vi "Master_DARPA.vi"() -> ()   [LabVIEW 2021]
uses:
  Control 2.ctl
  Settings.ctl
  <vilib>/DAQmx/write.llb/DAQmx Write (Analog DBL 1Chan 1Samp).vi
  <vilib>/DAQmx/write.llb/DAQmx Write (Analog Wfm 1Chan NSamp).vi
  <vilib>/DAQmx/write.llb/DAQmx Write (Digital 1D U32 1Chan NSamp).vi
  <vilib>/DAQmx/read.llb/DAQmx Read (Counter DBL 1Chan 1Samp).vi
  <vilib>/DAQmx/create/channels.llb/DAQmx Create Channel (AO-Voltage-Basic).vi
  <vilib>/DAQmx/create/channels.llb/DAQmx Create Channel (CI-Count Edges).vi
  <vilib>/DAQmx/miscellaneous.llb/DAQmx Fill In Error Info.vi
  <vilib>/DAQmx/create/channels.llb/DAQmx Create Channel (DO-Digital Output).vi
  <vilib>/DAQmx/configure/timing.llb/DAQmx Timing (Sample Clock).vi
  <resource>/objmgr/daqmx.rc
panel:
  out "s per ch":T1 format="%#_9f"
  out "Trial End Signal":bool
  in  "stop":bool
  in  "Blue Exposure Width [50-100] (ms)":T1=41.0 format="%#_9f"
  in  "Amber Start Time":T1=60.0 format="%#_9f"
  in  "Red Start (ms)":T1=120.0 format="%#_9f"
  in  "Red Exposure Width (ms)":T1=41.0 format="%#_9f"
  in  "Amber Exposure Width (ms)":T1=41.0 format="%#_9f"
  in  "base path":path=path "E:/DARPA/MW-LSCI1/5_14_22"
  in  "Delay end (ms)":dbl=102.0
  out "Stimulation":bool
  in  "AOM Voltage":dbl=0.085 format="%0.3f"
  out "String 7":string="AOM Settings"
  out "String 6":string="Stroke Settings"
  out "String 5":string="Intrinsic Imaging"
  in  "LED 625 nm":bool
  in  "LED 580 nm":bool
  out "Trial #":i32=2
  out "Frames acquired":dbl=576.0 format="%0.2f"
  out "Number of Samples (Total)":dbl=18000.0
  out "Period (ms)":dbl=6.5
  out "String 4":string="Experimental Summary"
  out "String 3":string="Stimulation Control"
  out "String 2":string="Sequence Control"
  out "String":string="Trials Control"
  in  "Strength (V)":dbl=10.0
  in  "# of stimulations":i32=2
  in  "Delay (ms)":dbl=35.0
  in  "Width of pulse (ms)":dbl=60.0
  in  "# of Sequences":dbl=750.0
  in  "Sampling Rate (Hz)":T1=100000.0 format="%#_9f"
  in  "Frames/Seq":i32=12
  in  "Exposure Width (ms)":T1=5.0 format="%#_9f"
  in  "Time Between (ms)":T2=1.5 format="%#_9f"
  in  "Pre-stimulus Time":dbl=30.0 format="%.6f"
  in  "Time b/w Trials (s)":dbl=10.0 caption="Delay Time (s)"
  in  "# Trials":i32=5
  in  "Time domain signal":T3(tab)
  out "LSCI Sequence":cluster{i32, dbl, dbl[]}(graph)={0, 1e-05, array[18000 elements]}
  out "Red LED":cluster{i32, dbl, dbl[]}(graph)={0, 1e-05, array[18000 elements]}
  out "Amber LED":cluster{i32, dbl, dbl[]}(graph)={0, 1e-05, array[18000 elements]}
  out "Blue LED":cluster{i32, dbl, dbl[]}(graph)={0, 1e-05, array[18000 elements]}
  out "EMCCD":cluster{i32, dbl, dbl[]}(graph)={0, 1e-05, array[18000 elements]}
  out "Whisker Cam":cluster{i32, dbl, dbl[]}(graph)={0, 1e-05, array[18000 elements]}
  out "Whisker Stim":cluster{i32, dbl, dbl[]}(graph)={0, 1e-05, array[18000 elements]}
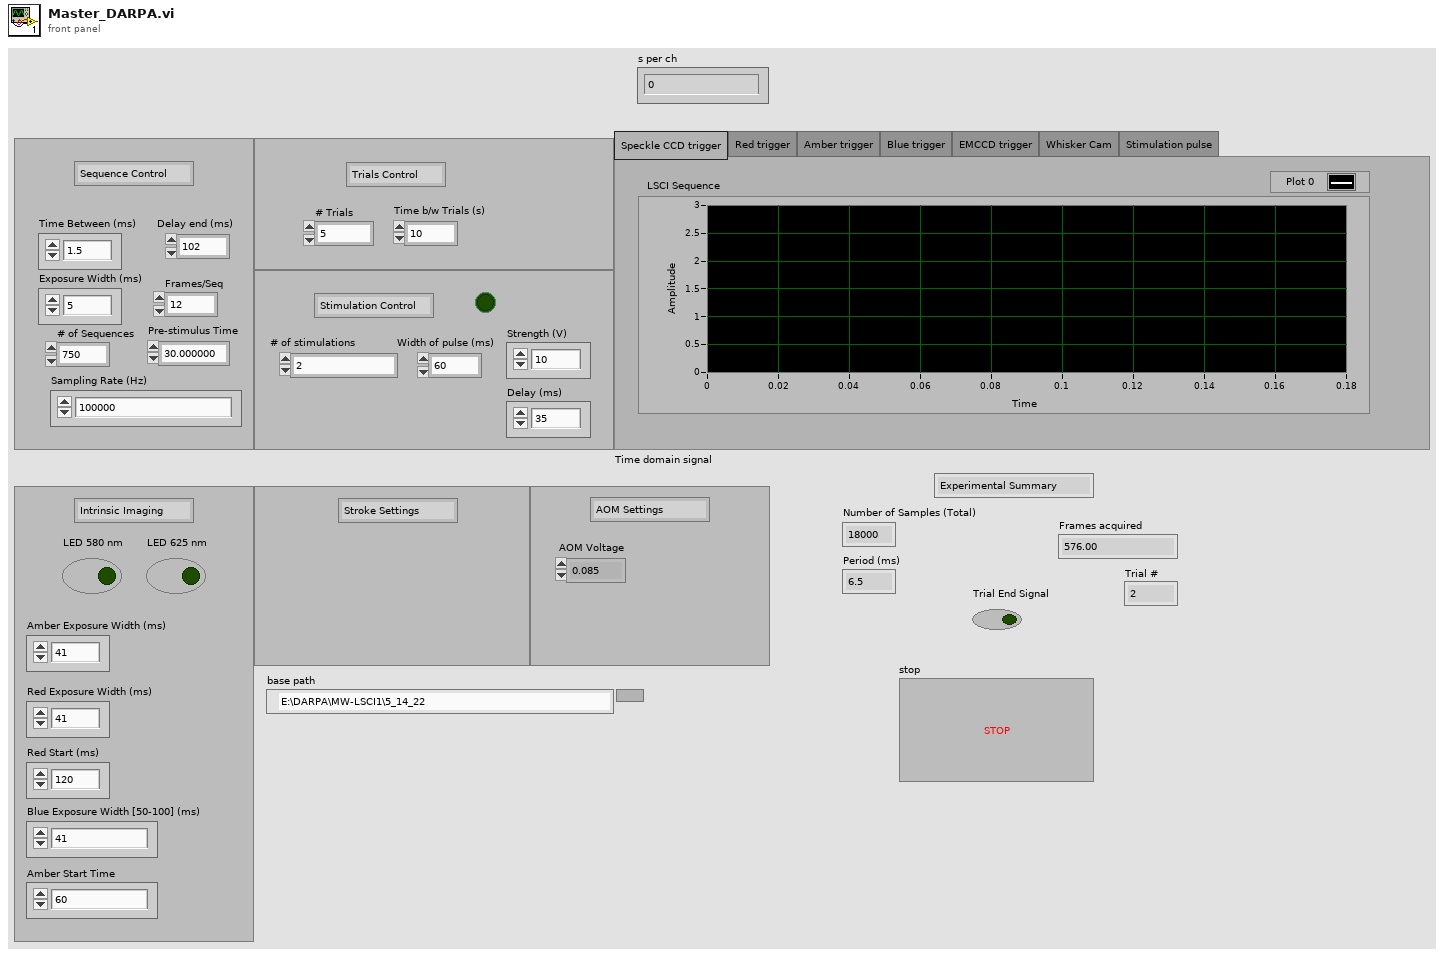
[diagram p1: front panel]
types:
  T1 = typedef "Settings.ctl" = dbl
  T2 = typedef "Control 2.ctl" = dbl
  T3 = enum32{"Speckle CCD trigger", "Red trigger", "Amber trigger", "Blue trigger", "EMCCD trigger", "Whisker Cam", "Stimulation pulse"}
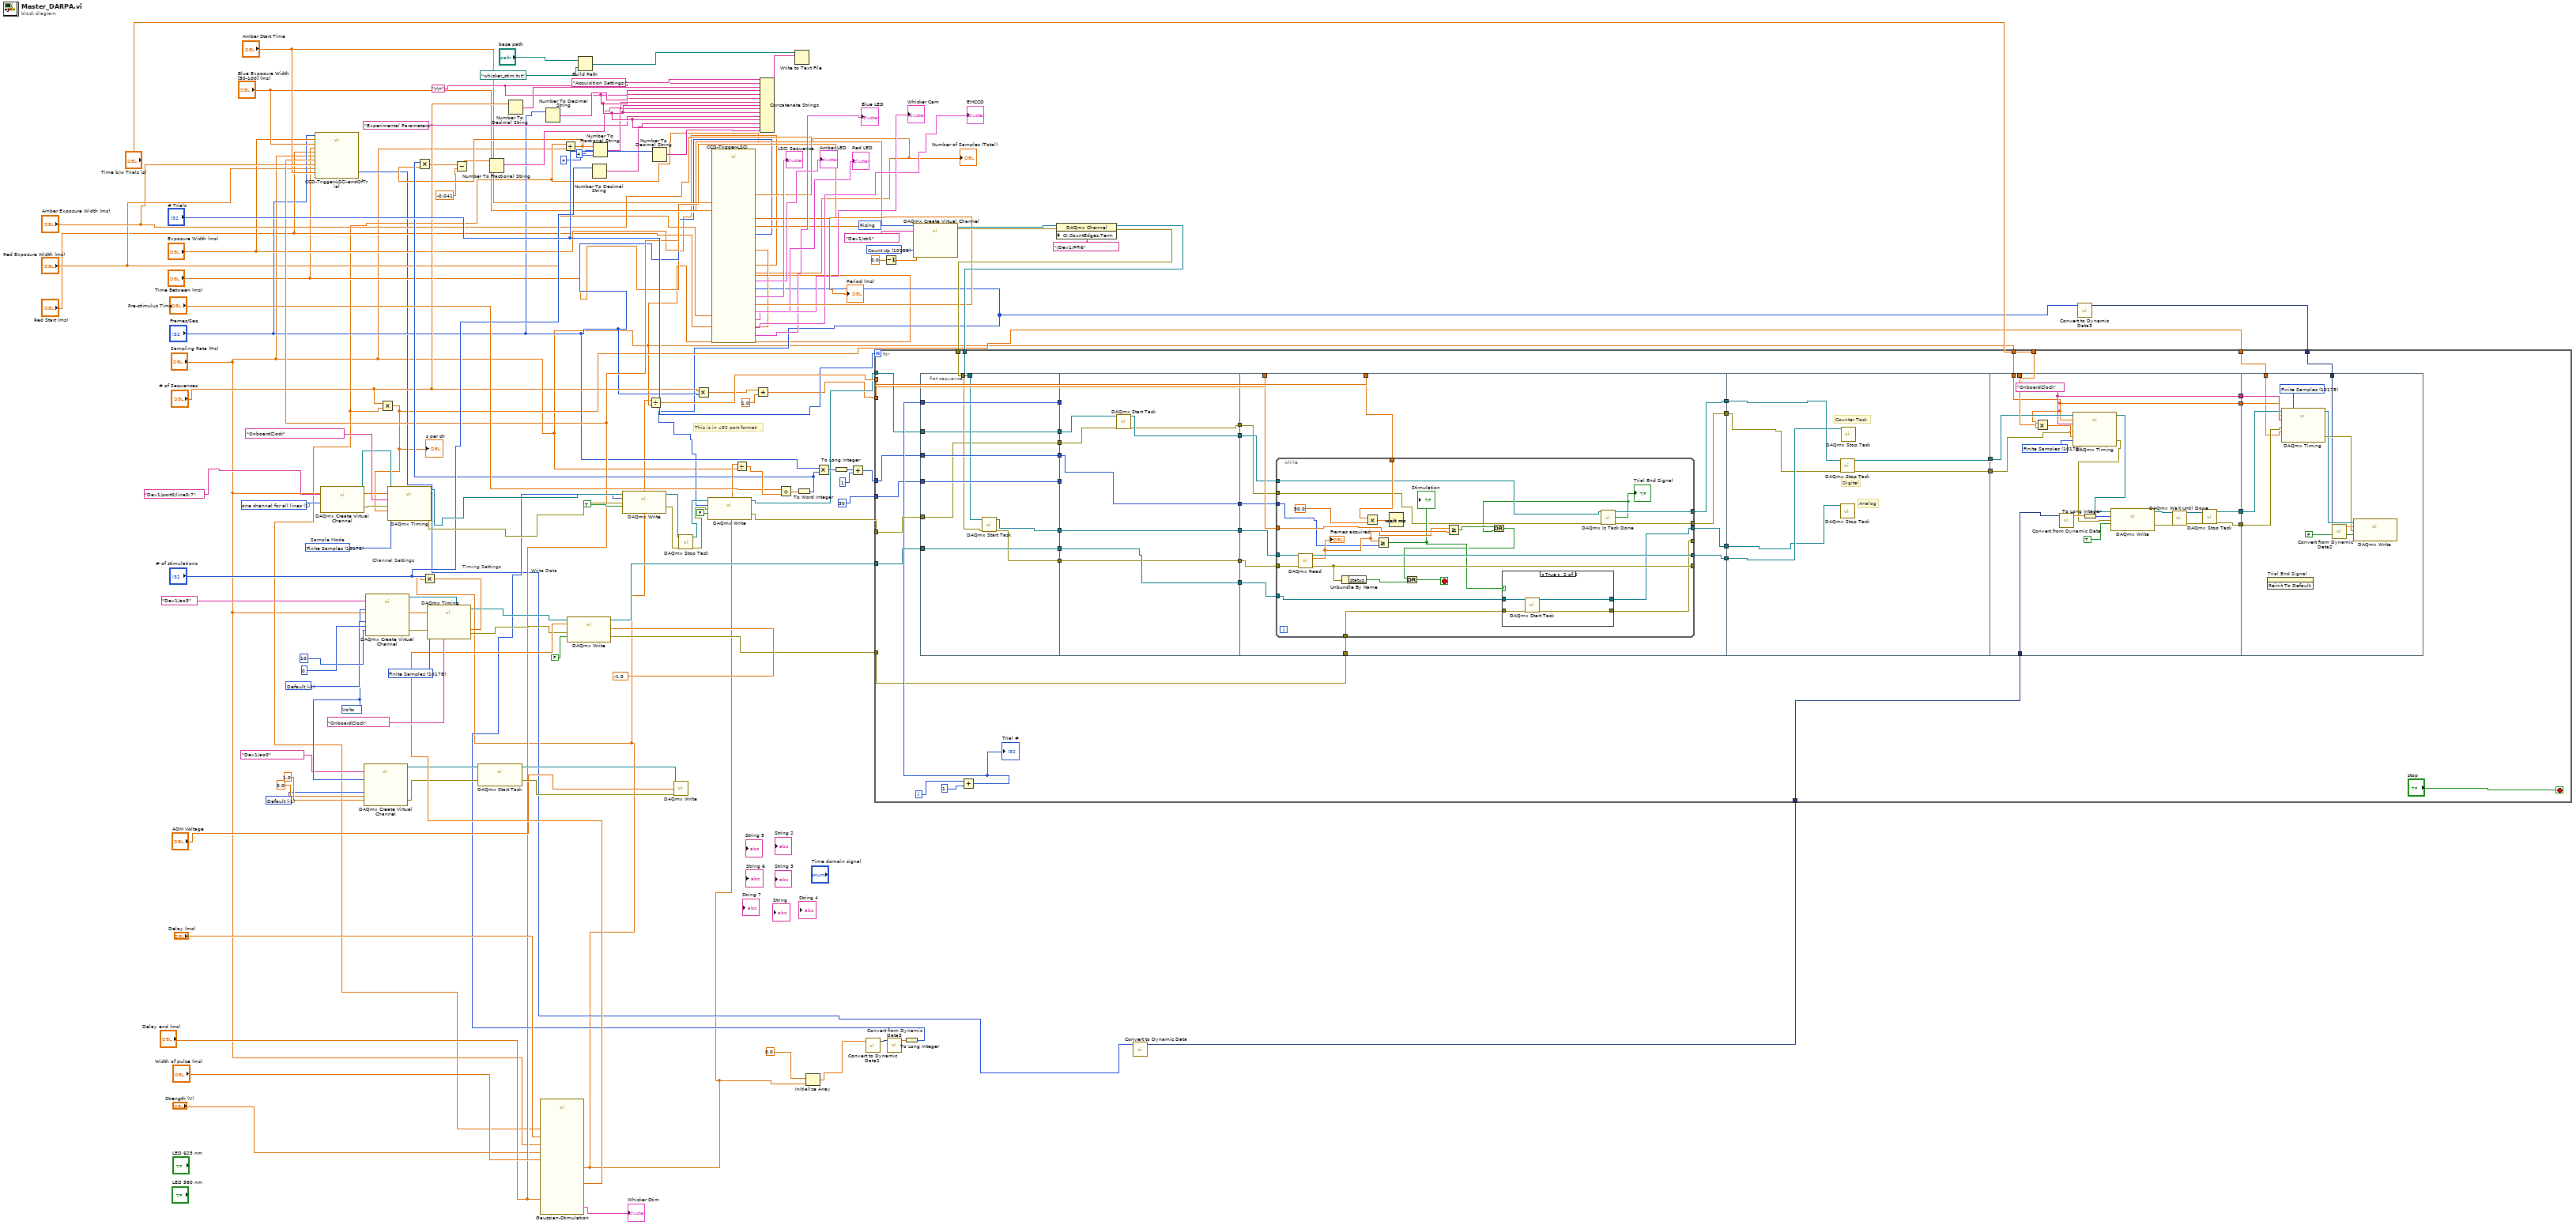
[diagram p0: block diagram]
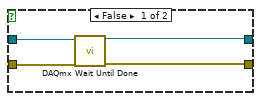
[diagram p2: hidden frame]
diagram:
  w63 = "\r\n"
  w73 = 1 items=["one channel for each line", "one channel for all lines"] ("line grouping")
  w88 = -1 items=["Default"=-1, "RSE"=10083, "Differential"=10106, "Pseudodifferential"=12529] ("output terminal configuration")
  w98 = 10280 items=["Rising"=10280, "Falling"=10171] ("edge")
  w102 = 10128 items=["Count Up"=10128, "Count Down"=10124, "Externally Controlled"=10326] ("count direction")
  w115 = 10178 items=["Finite Samples"=10178, "Continuous Samples"=10123] ("sample mode")
  w116 = -1 items=["Default"=-1, "RSE"=10083, "Differential"=10106, "Pseudodifferential"=12529] ("output terminal configuration")
  w90 = 10348 items=["Volts"=10348, "From Custom Scale"=10065] ("units")
  w121 = 10178 items=["Finite Samples"=10178, "Continuous Samples"=10123, "Hardware Timed Single Point"=12522]  # Sample Mode
  # "This is in u32 port format"
  # "Timing Settings"
  # "Write Data"
  # "Channel Settings"
  n1 = call "CCD-Trigger-LSCI-endOfTrial.vi"("Frames/Seq"="Frames/Seq", "Exposure Width (ms) in"="Exposure Width (ms)", "Blue Exposure Width [50-100] (ms)"="Blue Exposure Width [50-100] (ms)", "Time Between (ms)"="Time Between (ms)", "Red Start Time"="Red Start (ms)", "Sampling Rate"="Sampling Rate (Hz)", "Amber Start Time"="Amber Start Time", "Red Exposure Width [50-80] (ms)"="Red Exposure Width (ms)", "Amber Exposure Width [50-100] (ms)"="Amber Exposure Width (ms)", "Delay End (ms)"="Delay end (ms)") -> ("Array out"=w12:u32[])  [unwired: 1 in, 8 out]
  n2 = call-poly <vilib>:"DAQmx Create Virtual Channel.vi"("lines"=tag "Dev1/port0/line0:7", "line grouping"=w73) -> ("task out"=w80:refnum<k21>, "error out"=w109:errorcluster)  [unwired: 12 in]
  n3 = call-poly <vilib>:"DAQmx Create Virtual Channel.vi"("maximum value"=1.0, "minimum value"=0.0, "output terminal configuration"=w88, "physical channels"=tag "Dev1/ao0", "units"=w90) -> ("task out"=w86:refnum<k21>, "error out"=w85:errorcluster)  [unwired: 9 in]
  n4 = call-poly <vilib>:"DAQmx Create Virtual Channel.vi"("maximum value"=10, "minimum value"=0, "output terminal configuration"=w116, "physical channels"=tag "Dev1/ao3", "units"=w90) -> ("task out"=w113:refnum<k21>, "error out"=w114:errorcluster)  [unwired: 9 in]
  n5 = call <vilib>:"DAQmx Start Task.vi"("task/channels in"=w86, "error in"=w85) -> ("task out"=w84:refnum<k21>, "error out"=w83:errorcluster)  [unwired: 12 in]
  n6 = Number To Decimal String(number="# of Sequences") -> (decimal integer string=w65:string)  [unwired: 1 in]
  n7 = Number To Decimal String(number="Frames/Seq") -> (decimal integer string=w64:string)  [unwired: 1 in]
  n8 = Build Path(base path="base path", name or relative path=path "whisker_stim.txt" ("default name")) -> (appended path=w67:path)
  n9 = Number To Decimal String(number="# of stimulations") -> (decimal integer string=w58:string)  [unwired: 1 in]
  n10 = Number To Decimal String(number="# Trials") -> (decimal integer string=w62:string)  [unwired: 1 in]
  n11 = call-poly <vilib>:"DAQmx Write.vi"("task/channels in"=w84, "data"="AOM Voltage", "error in"=w83) -> ()  [unwired: 10 in, 3 out]
  n12 = Multiply(x="# of Sequences", y="Frames/Seq") -> (x*y=w15:dbl)
  n13 = call "CCD-Trigger-LSCI.vi"("Frames/Seq"="Frames/Seq", "Exposure Width (ms) in"="Exposure Width (ms)", "Blue Exposure Width [50-100] (ms)"="Blue Exposure Width [50-100] (ms)", "Time Between (ms)"="Time Between (ms)", "Red Start Time"="Red Start (ms)", "Sampling Rate"="Sampling Rate (Hz)", "Amber Start Time"="Amber Start Time", "Red Exposure Width [50-80] (ms)"="Red Exposure Width (ms)", "Amber Exposure Width [50-100] (ms)"="Amber Exposure Width (ms)", "Delay End (ms)"="Delay end (ms)") -> ("Blue LED"=→"Blue LED":cluster{i32, dbl, dbl[]}, "LSCI CCD"=→"LSCI Sequence":cluster{i32, dbl, dbl[]}, "Amber LED"=→"Amber LED":cluster{i32, dbl, dbl[]}, "Whisker Cam"=→"Whisker Cam":cluster{i32, dbl, dbl[]}, "EMCCD Trigger"=→"EMCCD":cluster{i32, dbl, dbl[]}, "Array out"=w9:u32[], "Period (ms)"=→"Period (ms)":dbl, "# Samples"=w4:T1, "Red LED"=→"Red LED":cluster{i32, dbl, dbl[]})  [unwired: 1 in]
  "Number of Samples (Total)" <- w4
  n14 = Multiply(x="# of Sequences", y=w4) -> (x*y=w10:T1)
  "s per ch" <- w10
  n15 = call-poly <vilib>:"DAQmx Timing.vi"("task/channels in"=w80, "sample mode"=w121, "samples per channel"=w10, "rate"="Sampling Rate (Hz)", "source"=tag "OnboardClock", "error in"=w109) -> ("task out"=w75:refnum<k21>, "error out"=w74:errorcluster)  [unwired: 8 in]
  n16 = call "Gaussian-Stimulation.vi"("Strength (V)"="Strength (V)", "Delay (ms)"="Delay (ms)", "# Samples in"=w4, "Delay end (ms)"="Delay end (ms)", "Width of pulse (ms)"="Width of pulse (ms)", "Sampling Rate"="Sampling Rate (Hz)") -> ("Array 2"=w106:T1[], "# Samples out"=w1:T1, "LSCI CCD"=→"Whisker Stim":cluster{i32, dbl, dbl[]})  [unwired: 1 in, 2 out]
  n17 = Multiply(x="# of stimulations", y=w1) -> (x*y=w110:T1)
  n18 = call-poly <vilib>:"DAQmx Timing.vi"("task/channels in"=w113, "sample mode"=w115, "samples per channel"=w110, "rate"="Sampling Rate (Hz)", "source"=tag "OnboardClock", "error in"=w114) -> ("task out"=w77:refnum<k21>, "error out"=w76:errorcluster)  [unwired: 1 in, 7 out]
  n19 = Divide(x=w4, y="Sampling Rate (Hz)") -> (x/y=w47:T1)
  n20 = call-poly <vilib>:"DAQmx Write.vi"("task/channels in"=w77, "auto start"=FALSE, "data"=w106, "timeout"=-1.0 ("Wirite Timeout"), "error in"=w76) -> ("task out"=w81:refnum<k21>, "error out"=w95:errorcluster)  [unwired: 9 out]
  n21 = Number To Fractional String(number=w47, width (-)=i16 4, precision (6)=i16 4) -> (F-format string=w57:string)  [unwired: 1 in]
  n22 = Divide(x=w1, y="Sampling Rate (Hz)") -> (x/y=w94:T1)
  n23 = Divide(x=w1, y="Sampling Rate (Hz)") -> (x/y=w72:T1)
  n24 = Add(x=w15, y=1.0) -> (x+y=w13:dbl)
  n25 = Divide(x="Pre-stimulus Time", y=w72) -> (x/y=w51:T1)
  n26 = To Word Integer(number=w51) -> (16bit integer=w50:i16)
  n27 = Multiply(x=w50, y=w47) -> (x*y=w6:T1)
  n28 = Subtract(x=w6, y=-0.041) -> (x-y=w7:T1)
  n29 = Number To Fractional String(number=w7) -> (F-format string=w54:string)  [unwired: 3 in]
  n30 = Concatenate Strings("Acquisition Settings:" ("string"), w63, w65, w63, w64, w63, w54, w63, w57, w63, "Experimental Parameters:" ("string"), w63, w58, w63, w62) -> (w61:string)
  n31 = Write to Text File(file (use dialog)=w67, text=w61) -> ()  [unwired: 2 in, 3 out]
  n32 = Initialize Array(0.0 ("element"), w1) -> (w16:dbl[])
  n33 = Multiply(x="Frames/Seq", y=w50) -> (x*y=w52:i32)
  n34 = To Long Integer(number=w52) -> (32bit integer=w46:i32)
  n35 = Add(x=w46, y=1) -> (x+y=w44:i32)
  n36 = call "Convert to Dynamic Data2"("Array"=w16) -> ("Dynamic Data Type"=w35:dynamicdata)  [unwired: 3 in]
  n37 = Decrement(x=0.0) -> (x-1=w101:dbl)
  n38 = call "Convert from Dynamic Data3"("Dynamic Data Type"=w35) -> ("Array"=w34:dbl[])  [unwired: 3 in]
  n39 = To Long Integer(number=w34) -> (32bit integer=w33:i32[])
  n40 = call-poly <vilib>:"DAQmx Write.vi"("task/channels in"=w75, "auto start"=TRUE, "data"=w33, "error in"=w74) -> ("task out"=w29:refnum<k21>, "error out"=w27:errorcluster)  [unwired: 9 in, 1 out]
  n41 = call <vilib>:"DAQmx Stop Task.vi"("task/channels in"=w29, "error in"=w27) -> ("task out"=w28:refnum<k21>, "error out"=w26:errorcluster)  [unwired: 12 in]
  n42 = call-poly <vilib>:"DAQmx Write.vi"("task/channels in"=w28, "auto start"=FALSE, "data"=w9, "error in"=w26) -> ("task out"=w30:refnum<k21>, "error out"=w31:errorcluster)  [unwired: 9 in, 1 out]
  n43 = call-poly <vilib>:"DAQmx Create Virtual Channel.vi"("initial count"=w101, "count direction"=w102, "edge"=w98, "counter"=tag "Dev1/ctr1") -> ("task out"=w99:refnum<k21>, "error out"=w100:errorcluster)  [unwired: 10 in]
  n44 = property class="DAQmx Channel"(reference=w99, error in=w100, "CI.CountEdges.Term"=tag "/Dev1/PFI6") -> (reference out=w70:refnum<k21>, error out=w71:errorcluster)
  n45 = call "Convert to Dynamic Data"("Array"=w12) -> ("Dynamic Data Type"=w11:dynamicdata)  [unwired: 3 in]
  n46 = call "Convert to Dynamic Data3"("Array"=w9) -> ("Dynamic Data Type"=w8:dynamicdata)  [unwired: 3 in]
  n47 = for {
    N: "# Trials" -> [_]
    tunnel: w31 -> [w164]
    tunnel: w81 -> [w163]
    tunnel: w95 -> [w149]
    tunnel: w30 -> [w151]
    tunnel: w94 -> [w162]
    tunnel: w13 -> [w135]
    tunnel: "Time b/w Trials (s)" -> [w131]
    tunnel: u32 30 ("Frames Per Second") -> [w158]
    tunnel: w71 -> [w142]
    tunnel: w70 -> [w141]
    tunnel: w44 -> [w136]
    tunnel: w11 -> [w130]
    tunnel: w10 -> [w124]
    tunnel: w8 -> [w123]
    tunnel: "Sampling Rate (Hz)" -> [w122]
    i -> [w161]
    stop <- "stop" stop-if-true
    n48 = flat-sequence {
      tunnel: w158 -> [w172]
      tunnel: w159 -> [w173]
      tunnel: w163 -> [w174]
      tunnel: w164 -> [w165]
      tunnel: [w165] -> w155
      tunnel: [w174] -> w154
      tunnel: [w173] -> w153
      tunnel: [w172] -> w152
      tunnel: w151 -> [w166]
      tunnel: [w166] -> w150
      tunnel: [w171] -> w147
      tunnel: w136 -> [w171]
      tunnel: w142 -> [w170]
      tunnel: w141 -> [w169]
      tunnel: [w168] -> w139
      tunnel: [w167] -> w138
      tunnel: w155 -> [w177]
      tunnel: w154 -> [w182]
      tunnel: w153 -> [_]
      tunnel: w152 -> [_]
      tunnel: w150 -> [w178]
      tunnel: [w176] -> w146
      tunnel: [w182] -> w145
      tunnel: [w181] -> w144
      tunnel: w147 -> [w181]
      tunnel: [w180] -> w140
      tunnel: w139 -> [w180]
      tunnel: w138 -> [w179]
      tunnel: [w179] -> w137
      tunnel: [w175] -> w134
      tunnel: w162 -> [w195]
      tunnel: w135 -> [w194]
      tunnel: [w193] -> w157
      tunnel: [w184] -> w156
      tunnel: w146 -> [w186]
      tunnel: w149 -> [w192]
      tunnel: w145 -> [w191]
      tunnel: [w190] -> w148
      tunnel: w144 -> [w189]
      tunnel: [w183] -> w143
      tunnel: w140 -> [w188]
      tunnel: w137 -> [w187]
      tunnel: w134 -> [w185]
      tunnel: w157 -> [w232]
      tunnel: w156 -> [w233]
      tunnel: w148 -> [w231]
      tunnel: w143 -> [w230]
      tunnel: [w229] -> w132
      tunnel: [w228] -> w129
      tunnel: w132 -> [w249]
      tunnel: w131 -> [w250]
      tunnel: w130 -> [w246]
      tunnel: w129 -> [w248]
      tunnel: [w235] -> w128
      tunnel: [w241] -> w127
      tunnel: [w238] -> w126
      tunnel: [w234] -> w125
      tunnel: w122 -> [w238]
      tunnel: w128 -> [w261]
      tunnel: w127 -> [w263]
      tunnel: w126 -> [w262]
      tunnel: w125 -> [w260]
      tunnel: w124 -> [w259]
      tunnel: w123 -> [w255]
      frame #0 {
        n49 = call <vilib>:"DAQmx Start Task.vi"("task/channels in"=w169, "error in"=w170) -> ("task out"=w168:refnum<k21>, "error out"=w167:errorcluster)  [unwired: 12 in]
      }
      frame #1 {
        n50 = call <vilib>:"DAQmx Start Task.vi"("task/channels in"=w178, "error in"=w177) -> ("task out"=w176:refnum<k21>, "error out"=w175:errorcluster)  [unwired: 12 out]
      }
      frame #2 {
        n51 = while {
          tunnel: w188 -> [w219]
          tunnel: w187 -> [w218]
          tunnel: [w217] -> w193
          tunnel: [w216] -> _
          tunnel: w195 -> [w215]
          tunnel: w194 -> [w208]
          tunnel: w192 -> [w211]
          tunnel: w191 -> [w212]
          tunnel: [w209] -> w190
          tunnel: [w210] -> _
          tunnel: w189 -> [w204]
          tunnel: w186 -> [w202]
          tunnel: w185 -> [w201]
          tunnel: [w200] -> w184
          tunnel: [w199] -> w183
          stop <- w205 stop-if-true
          n52 = call-poly <vilib>:"DAQmx Read.vi"("task/channels in"=w219, "error in"=w218) -> ("task out"=w217:refnum<k21>, "data"=w207:dbl, "error out"=w216:errorcluster)  [unwired: 11 in]
          "Frames acquired" <- w207
          n53 = Unbundle By Name(w216) -> ("status"=w206:bool)
          n54 = Multiply(x=w215, y=T1 50.0) -> (x*y=w214:T1)
          n55 = Greater Or Equal?(x=w207, y=w204) -> (x >= y?=w203:bool)
          "Stimulation" <- w203
          n56 = Wait (ms)(milliseconds to wait=w214) -> ()  [unwired: 1 out]
          n57 = Greater Or Equal?(x=w207, y=w208) -> (x >= y?=w198:bool)
          n58 = case shown="True" w203 {
            tunnel: w212 -> [w223 w227]
            tunnel: w211 -> [w222 w226]
            tunnel: [w220 w225] -> w210
            tunnel: [w221 w224] -> w209
            frame False {
              n59 = call <vilib>:"DAQmx Wait Until Done.vi"("task/channels in"=w223, "error in"=w222) -> ("task out"=w221:refnum<k21>, "error out"=w220:errorcluster)  [unwired: 12 in]
            }
            frame True {
              n60 = call <vilib>:"DAQmx Start Task.vi"("task/channels in"=w227, "error in"=w226) -> ("task out"=w224:refnum<k21>, "error out"=w225:errorcluster)  [unwired: 12 out]
            }
          }
          n61 = call <vilib>:"DAQmx Is Task Done.vi"("task/channels in"=w202, "error in"=w201) -> ("task out"=w200:refnum<k21>, "task done?"=w197:bool, "error out"=w199:errorcluster)  [unwired: 11 in]
          "Trial End Signal" <- w197
          n62 = Or(x=w198, y=w197) -> (x .or. y?=w196:bool)
          n63 = Or(x=w196, y=w206) -> (x .or. y?=w205:bool)
        }
      }
      frame #3 {
        # "Analog"
        # "Digital"
        # "Counter Task"
        n64 = call <vilib>:"DAQmx Stop Task.vi"("task/channels in"=w233, "error in"=w230) -> ("task out"=w229:refnum<k21>, "error out"=w228:errorcluster)  [unwired: 12 in]
        n65 = call <vilib>:"DAQmx Stop Task.vi"("task/channels in"=w231) -> ()  [unwired: 13 in, 2 out]
        n66 = call <vilib>:"DAQmx Stop Task.vi"("task/channels in"=w232) -> ()  [unwired: 13 in, 2 out]
      }
      frame #4 {
        w241 = tag "OnboardClock" ("source")
        w252 = 10178 items=["Finite Samples"=10178, "Continuous Samples"=10123, "Hardware Timed Single Point"=12522] ("sample mode")
        n67 = Multiply(x=w238, y=w250) -> (x*y=w251:T1)
        n68 = call "Convert from Dynamic Data"("Dynamic Data Type"=w246) -> ("Array"=w245:dbl[])  [unwired: 3 in]
        n69 = call-poly <vilib>:"DAQmx Timing.vi"("task/channels in"=w249, "sample mode"=w252, "samples per channel"=w251, "rate"=w238, "source"=w241, "error in"=w248) -> ("task out"=w247:refnum<k21>, "error out"=w243:errorcluster)  [unwired: 8 in]
        n70 = To Long Integer(number=w245) -> (32bit integer=w244:i32[])
        n71 = call-poly <vilib>:"DAQmx Write.vi"("task/channels in"=w247, "auto start"=TRUE, "data"=w244, "error in"=w243) -> ("task out"=w240:refnum<k21>, "error out"=w239:errorcluster)  [unwired: 9 in, 1 out]
        n72 = call <vilib>:"DAQmx Wait Until Done.vi"("task/channels in"=w240, "error in"=w239) -> ("task out"=w237:refnum<k21>, "error out"=w236:errorcluster)  [unwired: 12 in]
        n73 = call <vilib>:"DAQmx Stop Task.vi"("task/channels in"=w237, "error in"=w236) -> ("task out"=w235:refnum<k21>, "error out"=w234:errorcluster)  [unwired: 12 in]
      }
      frame #5 {
        w258 = 10178 items=["Finite Samples"=10178, "Continuous Samples"=10123, "Hardware Timed Single Point"=12522] ("sample mode")
        n74 = invoke on="Trial End Signal" class="Bool (strict)" method="Reinit To Default"() -> ()  [unwired: 3 in, 3 out]
        n75 = call-poly <vilib>:"DAQmx Timing.vi"("task/channels in"=w261, "sample mode"=w258, "samples per channel"=w259, "rate"=w262, "source"=w263, "error in"=w260) -> ("task out"=w257:refnum<k21>, "error out"=w256:errorcluster)  [unwired: 8 in]
        n76 = call "Convert from Dynamic Data2"("Dynamic Data Type"=w255) -> ("Array"=w254:dbl[])  [unwired: 3 in]
        n77 = call-poly <vilib>:"DAQmx Write.vi"("task/channels in"=w257, "auto start"=FALSE, "data"=w254, "error in"=w256) -> ()  [unwired: 9 in, 3 out]
      }
    }
    n78 = Add(x=w161, y=1) -> (x+y=w159:i32)
    "Trial #" <- w159
  }
